vi "Init Panels.vi"(8 "error in (no error)":errorcluster, 11 "SB App in":refnum<class "SB App.lvclass">) -> (0 "error out":errorcluster, 3 "SB App out":refnum<class "SB App.lvclass">)   [LabVIEW 2020, in "SB App.lvlib" / "SB App.lvclass"]
uses:
  SB App.lvclass
  Team Field Panel/Team Field Panel.lvclass
  C:/Program Files (x86)/National Instruments/LabVIEW 2020/vi.lib/IlluminatedG/IG OOPanel/OOPanel/Panel/Panel.lvclass
  Square Field Panel/Square Field Panel.lvclass
  SB App.lvclass/SB App.ctl
  <vilib>/IlluminatedG/IG OOPanel/OOPanel/Manager/Manager.lvclass
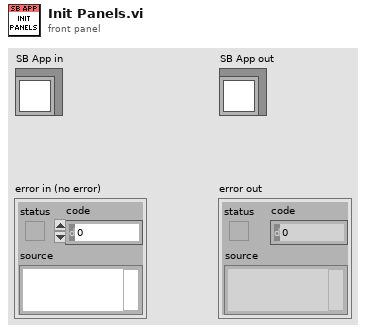
[diagram p1: front panel]
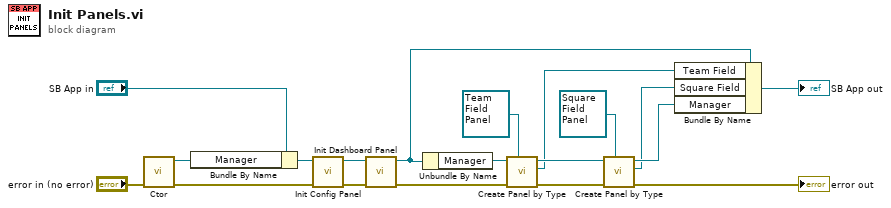
[diagram p0: block diagram]
diagram:
  n1 = call <vilib>:"Ctor.vi"("error in (no error)"="error in (no error)") -> ("error out"=w8:errorcluster, "Manager out"=w10:refnum<class "Manager.lvclass">)  [unwired: 9 in]
  n2 = Bundle By Name(cluster="SB App in", "Manager"=w10) -> (w7:refnum<class "SB App.lvclass">)
  n3 = call "Init Config Panel.vi"("error in (no error)"=w8, "SB App in"=w7) -> ("error out"=w5:errorcluster, "SB App out"=w6:refnum<class "SB App.lvclass">)  [unwired: 8 in]
  n4 = call "Init Dashboard Panel.vi"("error in (no error)"=w5, "SB App in"=w6) -> ("error out"=w3:errorcluster, "SB App out"=w2:refnum<class "SB App.lvclass">)  [unwired: 8 in]
  n5 = Unbundle By Name(w2) -> ("Manager"=w4:refnum<class "Manager.lvclass">)
  n6 = call <vilib>:"Create Panel by Type.vi"("Panel Type"=refnum<class "Team Field Panel.lvclass"> refnum ("SB App.lvlib:Team Field Panel.lvclass"), "error in (no error)"=w3, "Manager in"=w4) -> ("error out"=w12:errorcluster, "Panel"=w14:refnum<class "Team Field Panel.lvclass">, "Manager out"=w17:refnum<class "Manager.lvclass">)  [unwired: 6 in]
  n7 = call <vilib>:"Create Panel by Type.vi"("Panel Type"=refnum<class "Square Field Panel.lvclass"> refnum ("SB App.lvlib:Square Field Panel.lvclass"), "error in (no error)"=w12, "Manager in"=w17) -> ("error out"=→"error out":errorcluster, "Panel"=w15:refnum<class "Square Field Panel.lvclass">, "Manager out"=w16:refnum<class "Manager.lvclass">)  [unwired: 6 in]
  n8 = Bundle By Name(cluster=w2, "Team Field"=w14, "Square Field"=w15, "Manager"=w16) -> (→"SB App out":refnum<class "SB App.lvclass">)
